vi "midiinopen.vi"(4 "error in (no error)":errorcluster, 5 "value":refnum<user-event>, 7 "MIDI Input Device":i32) -> (0 "error out":errorcluster, 1 "value out":refnum<user-event>, 2 "output param":i32, 3 "hmidiin":i32)   [LabVIEW 2014]
doc: "Opens a reference to a MIDI Input Device and retrieves a \"value\" from a Windows callback using the \"MIDIDLL.dll\". The \"value\" is then available for the Event Structure."
uses:
  mididll.dll
panel:
  # "Input Data"
  # "Local Data"
  # "Output Data"
  # "No local data."
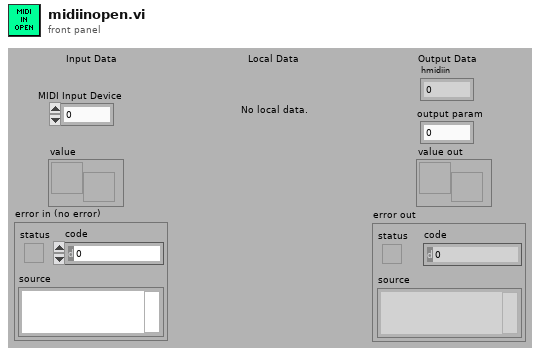
[diagram p1: front panel]
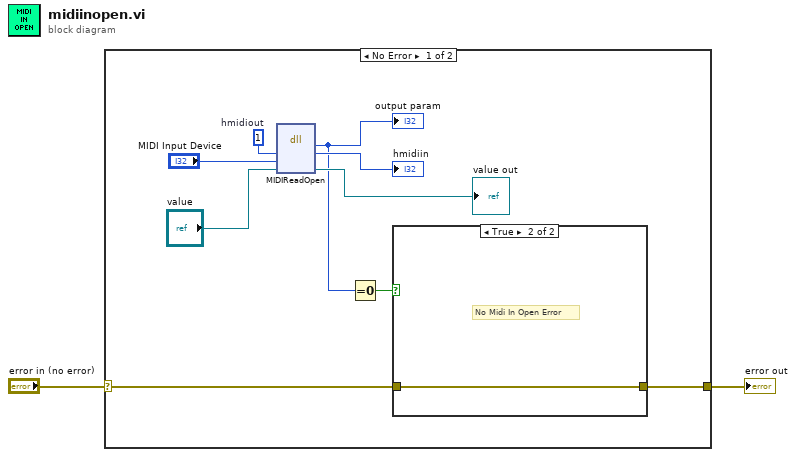
[diagram p0: block diagram]
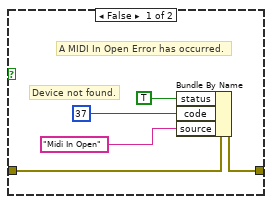
[diagram p2: hidden frame]
diagram:
  n1 = case shown="No Error" "error in (no error)" {
    selector: "error in (no error)" -> [w4 w18]
    tunnel: [w3 w18] -> w1
    frame No Error {
      w11 = 1  # hmidiout
      n2 = dll-call lib="C:/Users/jag2k2/Desktop/Flashcards/MIDI Throughput Release 1.0/LabVIEW Code/MIDIDLL.dll" fn="MIDIReadOpen"("hmidiin"=w11, "deviceID"="MIDI Input Device", "value"="value") -> (w5:i32, "hmidiin"=→"hmidiin":i32, "value"=→"value out":refnum<user-event>)  [unwired: 4 in, 2 out]
      "output param" <- w5
      n3 = Equal To 0?(x=w5) -> (x = 0?=w6:bool)
      n4 = case shown="True" w6 {
        tunnel: w4 -> [w16 w17]
        tunnel: [w15 w17] -> w3
        frame False {
          # "Device not found."
          # "A MIDI In Open Error has occurred."
          n5 = Bundle By Name(cluster=w16, "status"=TRUE, "code"=37, "source"="Midi In Open") -> (w15:errorcluster)
        }
        frame True {
          # "No Midi In Open Error"
        }
      }
    }
    frame Error {
    }
  }
  "error out" <- w1
